vi "Global - Configuration Options.vi"() -> ()   [LabVIEW 2018]
panel:
  in  "Error Log Path":path=path "c:/log/log.txt"
  in  "Data Log Folder":path=path "C:/data"
  in  "Network Stream Buffer Size":i32=50
  in  "Reboot Timestamp Log":path=path "c:/log/reboots.txt"
  in  "Error Log Duplicate Interval (ms)":u32=5000
  in  "Network Stream Polling Timeout (ms)":i32=500
  in  "Debugging":bool=TRUE
  in  "Error Log Max Size (bytes)":i64=100000
  in  "RT Stream Name":string="Command Stream from RT"
  in  "Monitoring Loop Rate (ms)":u32=200
  in  "UI Stream Name":string="Command Stream from UI"
  in  "Network Stream Connect Timeout (ms)":i32=5000
  # "If you change any of these default configuration options, you must select Edit > Make Current Values Default before saving this VI."
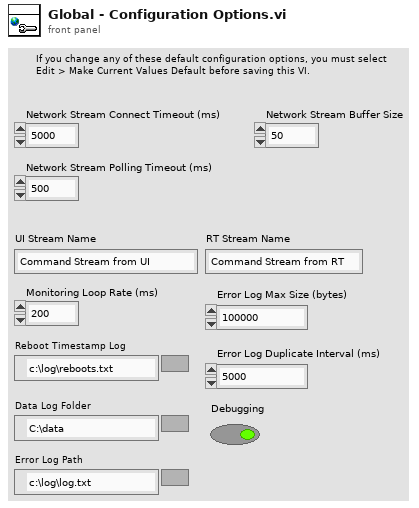
[diagram p1: front panel]
diagram:
